vi "init daq state.vi"(0 "T cont wait time (ms)":i32=200, 7 "DAQ clust in":T4={"DAQ state"=enum."Global comm", "temp"={"T exec"={"T mode"=enum."settling", "exec setpoint"=0.0, "reset"=FALSE, "man power"=0.0, "man"=FALSE, "log"=FALSE, "clear"=FALSE}, "T status"={"Control status"=enum."In Settle Band", "Temp"=0.0, "Power"=0.0, "Time in settle band"=0.0, "Settled"=FALSE, "Low"=FALSE, "High"=FALSE, "Setpoint"=0.0, "Control"=FALSE, "In Settle Band"=FALSE}, "T params"={"Setpoint"=0.0, "Control Bandwidth"=0.0, "Integral Time"=0.0, "Int\nON"=FALSE, "Derivative Tme"=0.0, "Der\nON"=FALSE, "Settle Bandwidth"=0.0, "Settle Time"=0.0}, "utility"={"meas index"=0, "wait (ms)"=0, "H Vmax"=0.0, "power out"=0.0, "heat volt out"=0.0, "heat volt in"=0.0, "therm volt"=0.0, "t T P hist"=[], "cont hist"=[]}}, "meas"={"wvfm params"={"Num of avg"=0, "Num points"=0, "Meas rate (Hz)"=0.0}, "avg"={"t0"=timestamp(0 s since 1904-01-01), "dt"=1.0, "Y"=[]}, "raw wvfms"=[], "progress"={"avg done"=FALSE, "meas index"=0, "N waves"=0}, "t (s)"=0.0}, "device"="Dev1", "error"={"status"=FALSE, "code"=0, "source"=""}, "start (ms)"=0} {"temp"."utility"."therm volt" format="%_6g"; "temp"."utility"."heat volt in" format="%_6g"; "temp"."utility"."heat volt out" format="%_6g"; "temp"."utility"."power out" format="%_6g"; "temp"."utility"."H Vmax" format="%_6g"; "temp"."T exec"."man power" format="%_6g"; "temp"."T exec"."exec setpoint" format="%_6g"; "temp"."T params"."Settle Time" step=1.0; "temp"."T params"."Settle Bandwidth" step=0.01; "temp"."T params"."Derivative Tme" step=0.01; "temp"."T params"."Integral Time" step=1.0; "temp"."T params"."Control Bandwidth" step=0.1; "temp"."T params"."Setpoint" step=0.1; "temp"."T status"."Setpoint" format="%_6g"; "temp"."T status"."Power" format="%_6g"; "temp"."T status"."Temp" format="%_6g"}, 11 "Default Setpoint (C)":dbl=30.0) -> (8 "DAQ clust out":T4={"DAQ state"=enum."Global comm", "temp"={"T exec"={"T mode"=enum."settling", "exec setpoint"=30.0, "reset"=FALSE, "man power"=0.0, "man"=FALSE, "log"=FALSE, "clear"=FALSE}, "T status"={"Control status"=enum."Below Control Band", "Temp"=nan, "Power"=nan, "Time in settle band"=0.0, "Settled"=FALSE, "Low"=TRUE, "High"=FALSE, "Setpoint"=30.0, "Control"=FALSE, "In Settle Band"=FALSE}, "T params"={"Setpoint"=30.0, "Control Bandwidth"=2.0, "Integral Time"=8.0, "Int\nON"=TRUE, "Derivative Tme"=0.1, "Der\nON"=TRUE, "Settle Bandwidth"=0.2, "Settle Time"=60.0}, "utility"={"meas index"=0, "wait (ms)"=250, "H Vmax"=8.5, "power out"=0.0, "heat volt out"=0.0, "heat volt in"=0.0, "therm volt"=0.0, "t T P hist"=[], "cont hist"=[]}}, "meas"={"wvfm params"={"Num of avg"=0, "Num points"=0, "Meas rate (Hz)"=0.0}, "avg"={"t0"=timestamp(0 s since 1904-01-01), "dt"=1.0, "Y"=[]}, "raw wvfms"=[], "progress"={"avg done"=FALSE, "meas index"=0, "N waves"=0}, "t (s)"=0.0}, "device"="Dev1", "error"={"status"=FALSE, "code"=0, "source"=""}, "start (ms)"=127493354} {"temp"."utility"."therm volt" format="%_6g"; "temp"."utility"."heat volt in" format="%_6g"; "temp"."utility"."heat volt out" format="%_6g"; "temp"."utility"."power out" format="%_6g"; "temp"."utility"."H Vmax" format="%_6g"; "temp"."T exec"."man power" format="%_6g"; "temp"."T exec"."exec setpoint" format="%_6g"; "temp"."T params"."Settle Time" step=1.0; "temp"."T params"."Settle Bandwidth" step=0.01; "temp"."T params"."Derivative Tme" step=0.01; "temp"."T params"."Integral Time" step=1.0; "temp"."T params"."Control Bandwidth" step=0.1; "temp"."T params"."Setpoint" step=0.1; "temp"."T status"."Setpoint" format="%_6g"; "temp"."T status"."Power" format="%_6g"; "temp"."T status"."Temp" format="%_6g"})   [LabVIEW 2019]
doc: "This is a Bug C(T) subVI.\n\nThis subvi initializes the temp daq state machine and the global variables for the bug experiment.\n\nPaul K Dixon\nP3600\nCSUSB Physics"
uses:
  typedefs/DAQ state cluster.ctl
  typedefs/DAQ state enum.ctl
  typedefs/temp cont cluster.ctl
  typedefs/temp exec cluster.ctl
  typedefs/temp mode enum.ctl
  typedefs/temp indicator.ctl
  typedefs/temp control status.ctl
  typedefs/PID control parameters.ctl
  typedefs/temp cont utility.ctl
  typedefs/measurement.ctl
  typedefs/wvfm acq params.ctl
  typedefs/result.ctl
  typedefs/cap fit params.ctl
  globals/Bug globals.vi
panel:
  in  "T cont.T status":T1={"Control status"=enum."Below Control Band", "Temp"=25.0, "Power"=0.0, "Time in settle band"=0.0, "Settled"=FALSE, "Low"=TRUE, "High"=FALSE, "Setpoint"=30.0, "Control"=FALSE, "In Settle Band"=FALSE} {"Setpoint" format="%_6g"; "Power" format="%_6g"; "Temp" format="%_6g"}
  in  "T cont.T params":T3={"Setpoint"=30.0, "Control Bandwidth"=1.0, "Integral Time"=10.0, "Int\nON"=TRUE, "Derivative Tme"=0.1, "Der\nON"=TRUE, "Settle Bandwidth"=0.2, "Settle Time"=60.0} {"Settle Time" step=1.0; "Settle Bandwidth" step=0.01; "Derivative Tme" step=0.01; "Integral Time" step=1.0; "Control Bandwidth" step=0.1; "Setpoint" step=0.1}
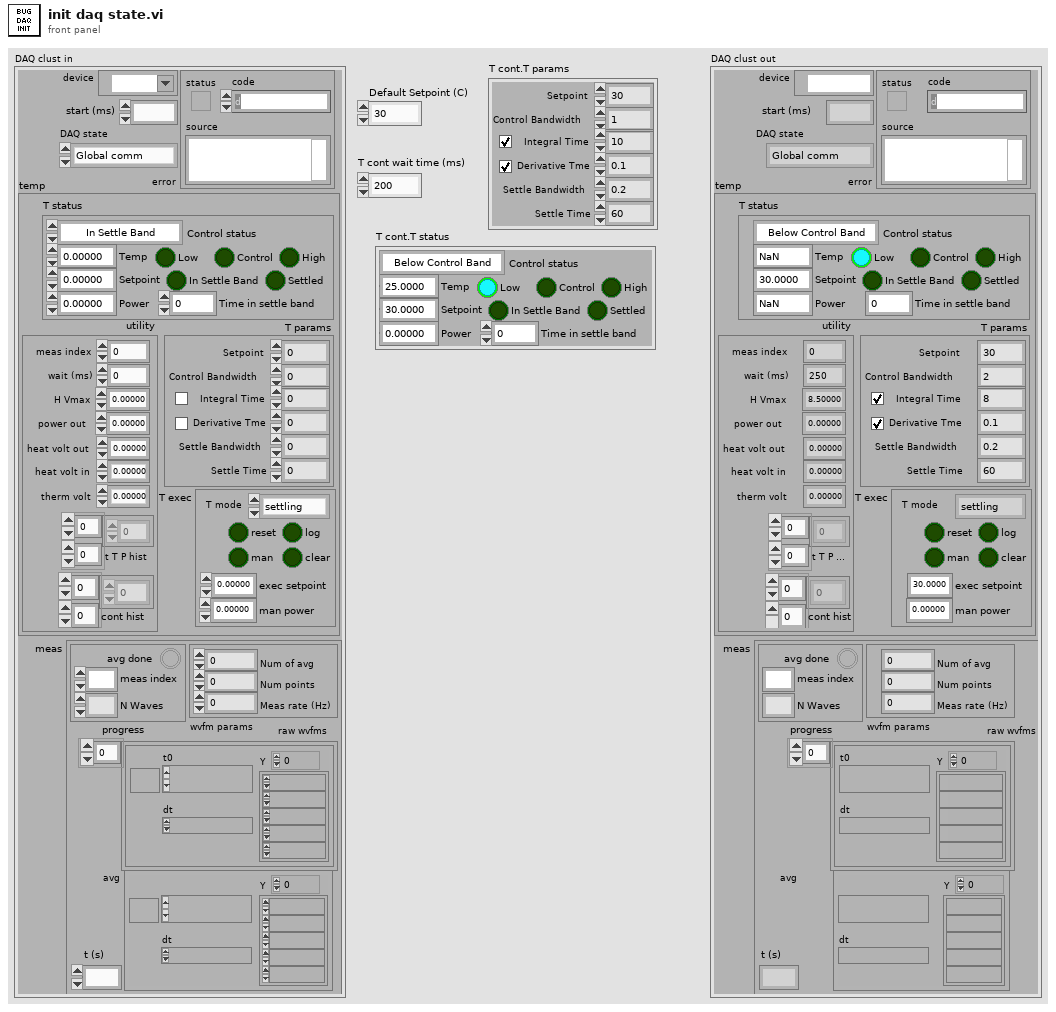
[diagram p1: front panel]
types:
  T1 = typedef "temp indicator.ctl" = cluster{"Control status":T2, "Temp":dbl, "Power":dbl, "Time in settle band":dbl, "Settled":bool, "Low":bool, "High":bool, "Setpoint":dbl, "Control":bool, "In Settle Band":bool}
  T2 = typedef "temp control status.ctl" = enum16{"In Settle Band", "In Control Band", "Below Control Band", "Above Control Band"}
  T3 = typedef "PID control parameters.ctl" = cluster{"Setpoint":dbl, "Control Bandwidth":dbl, "Integral Time":dbl, "Int\nON":bool, "Derivative Tme":dbl, "Der\nON":bool, "Settle Bandwidth":dbl, "Settle Time":dbl}
  T4 = typedef "DAQ state cluster.ctl" = cluster{"DAQ state":T5, "temp":T6, "meas":T10, "device":tag, "error":errorcluster, "start (ms)":i32}
  T5 = typedef "DAQ state enum.ctl" = enum16{"Global comm", "Meas T & P", "PID power calc", "Man Power set", "Output Power", "Wait", "Meas wvfm", "Avg wvfm", "Exit"}
  T6 = typedef "temp cont cluster.ctl" = cluster{"T exec":T7, "T status":T1, "T params":T3, "utility":T9}
  T7 = typedef "temp exec cluster.ctl" = cluster{"T mode":T8, "exec setpoint":dbl, "reset":bool, "man power":dbl, "man":bool, "log":bool, "clear":bool}
  T8 = typedef "temp mode enum.ctl" = enum16{"settling", "measuring", "holding", "Exit"}
  T9 = typedef "temp cont utility.ctl" = cluster{"meas index":i32, "wait (ms)":i32, "H Vmax":dbl, "power out":dbl, "heat volt out":dbl, "heat volt in":dbl, "therm volt":dbl, "t T P hist":dbl[][], "cont hist":dbl[][]}
  T10 = typedef "measurement.ctl" = cluster{"wvfm params":T11, "avg":waveform(dbl), "raw wvfms":waveform(dbl)[], "progress":cluster{"avg done":bool, "meas index":i32, "N waves":i32}, "t (s)":dbl}
  T11 = typedef "wvfm acq params.ctl" = cluster{"Num of avg":i32, "Num points":i32, "Meas rate (Hz)":dbl}
  T12 = typedef "result.ctl" = cluster{"Temp (C)":dbl, "RC Fit":T13, "wave":waveform(dbl), "Time (s)":dbl}
  T13 = typedef "cap fit params.ctl" = cluster{"Resistance (Ohms)":dbl, "Est Time constant (s)":dbl, "Est Capacitance (F)":dbl}
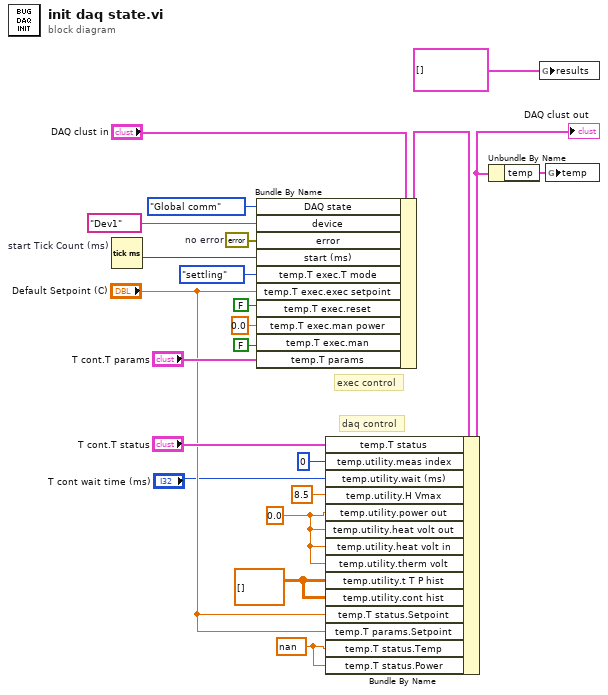
[diagram p0: block diagram]
diagram:
  w5 = nan ("T cont.T status.Temp")
  w9 = 0.0 ("T cont.H Vmax")
  w8 = dbl[][] [] ("T cont.T hist")
  w18 = errorcluster {"status"=FALSE, "code"=0, "source"=""}  # no error
  # "daq control"
  # "exec control"
  n1 = Tick Count (ms) "start Tick Count (ms)"() -> (millisecond timer value=w6:u32)
  n2 = Bundle By Name(cluster="DAQ clust in", "DAQ state"=DAQ_state_enum."Global comm", "device"=tag "Dev1", "error"=w18, "start (ms)"=w6, "temp.T exec.T mode"=temp_mode_enum."settling" ("T cont.exec.T mode"), "temp.T exec.exec setpoint"="Default Setpoint (C)", "temp.T exec.reset"=FALSE ("T cont.exec.reset"), "temp.T exec.man power"=0.0 ("T cont.exec.man power"), "temp.T exec.man"=FALSE ("T cont.exec.man"), "temp.T params"="T cont.T params") -> (w16:T4)
  n3 = Bundle By Name(cluster=w16, "temp.T status"="T cont.T status", "temp.utility.meas index"=0 ("T cont.therm volt"), "temp.utility.wait (ms)"="T cont wait time (ms)", "temp.utility.H Vmax"=8.5 ("T cont.H Vmax"), "temp.utility.power out"=w9, "temp.utility.heat volt out"=w9, "temp.utility.heat volt in"=w9, "temp.utility.therm volt"=w9, "temp.utility.t T P hist"=w8, "temp.utility.cont hist"=w8, "temp.T status.Setpoint"="Default Setpoint (C)", "temp.T params.Setpoint"="Default Setpoint (C)", "temp.T status.Temp"=w5, "temp.T status.Power"=w5) -> (w7:T4)
  "DAQ clust out" <- w7
  n4 = Unbundle By Name(w7) -> ("temp"=w2:T6)
  n5 = global write "Bug globals.vi" "results"(T12[] [] ("results")) -> ()
  n6 = global write "Bug globals.vi" "temp"(w2) -> ()
